vi "Modbus Master Example.vi"() -> ()   [LabVIEW 2018]
doc: "An example of the modbus master functionality."
uses:
  API/Wrapper/API Main.lvlib
  Master Function Definition/Read Device ID code.ctl
  Data Model/Device Data Model.lvclass
  API/Wrapper/Create TCP Master.vi
  API/Master/Modbus Master.lvclass
panel:
  out "element":refnum<vi>
  in  "index":i32
  in  "Stop Button":bool
  in  "Port":u16=502
  in  "Set Holding Registers":bool
  in  "Set Coils":bool
  in  "Fetch Discrete Inputs":bool
  in  "Fetch Input Registers":bool
  in  "Fetch Basic Objects":bool
  out "Basic Objects":string[](array[string])
  out "Status":string
  in  "Disconnect":bool
  in  "Connect":bool
  in  "Holding Registers":u16[](array[numeric])=[0, 0, 0, 0, 0, 0, 0, 0]
  out "Input Registers":u16[](array[numeric])
  in  "Coils":bool[](array[boolean])=[FALSE, FALSE, FALSE, FALSE, FALSE, FALSE, FALSE, FALSE]
  out "Discrete Inputs":bool[](array[boolean])
  in  "Slave Address":string="localhost"
  # "Coils are the boolean outputs of a modbus device. This example allows you to set the first 8 outputs."
  # "Holding Registers are the integer outputs of a modbus device. This example allows you to set the first 8 outputs."
  # "Modbus devices can also store objects in their memory, which are variable length strings. This example requests the basic level of objects."
  # "Discrete inputs are the boolean inputs of a modbus device. This example allows you to read the first 8 inputs."
  # "Input Registers are the integer inputs of a modbus device. This example allows you to read the first 8 inputs."
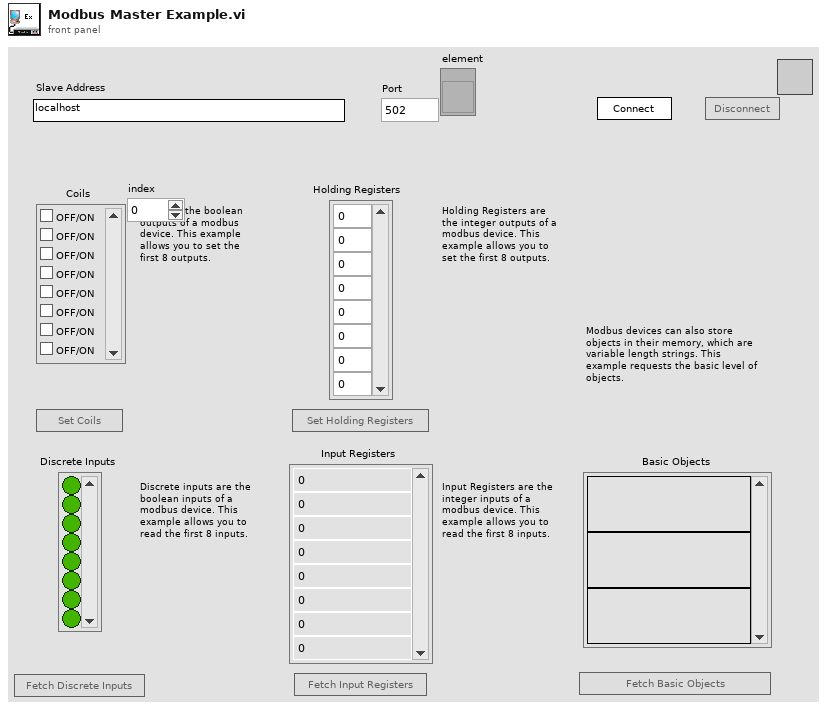
[diagram p1: front panel]
types:
  T1 = enum8{"Enabled", "Disabled", "Disabled and Grayed Out"}
  T2 = typedef "Device Data Model.lvclass/Read Device ID code.ctl" = enum8{"Read Basic", "Read Regular", "Read Extended", "Read Specific"}
  T3 = typedef "Device Data Model.lvclass/Identification Parameters.ctl" = cluster{"Object ID":u8, "Value":string}
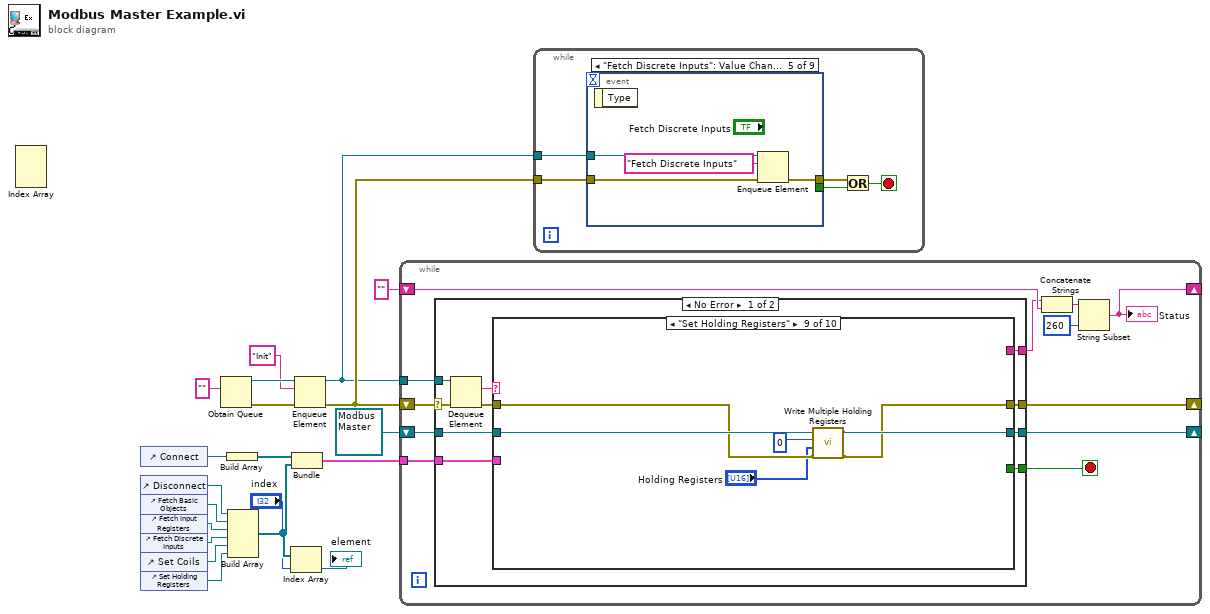
[diagram p0: block diagram]
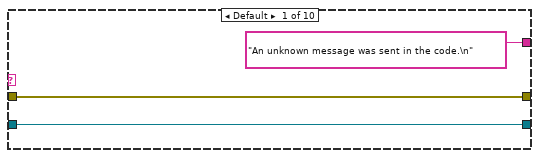
[diagram p2: hidden frame]
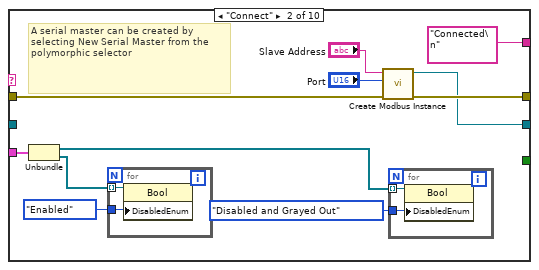
[diagram p3: hidden frame]
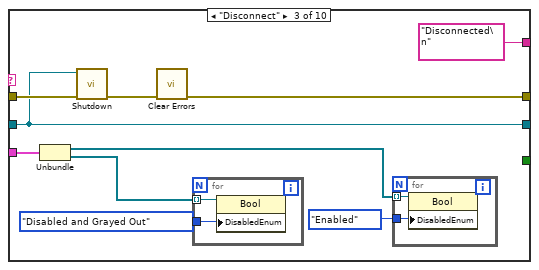
[diagram p4: hidden frame]
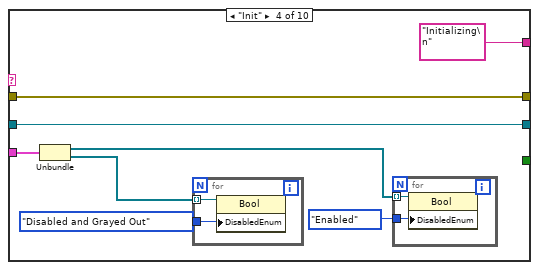
[diagram p5: hidden frame]
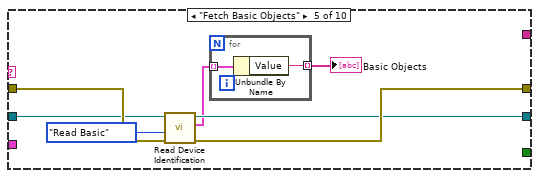
[diagram p6: hidden frame]
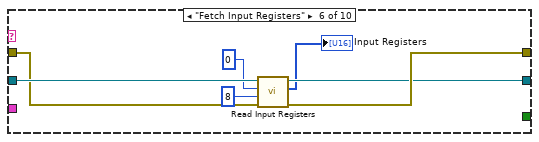
[diagram p7: hidden frame]
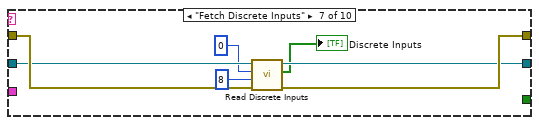
[diagram p8: hidden frame]
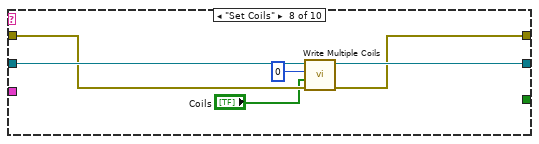
[diagram p9: hidden frame]
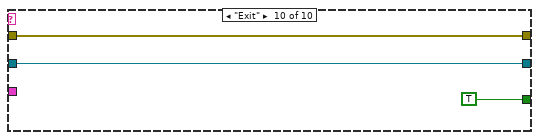
[diagram p10: hidden frame]
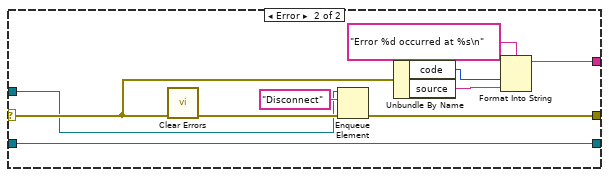
[diagram p11: hidden frame]
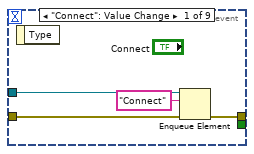
[diagram p12: hidden frame]
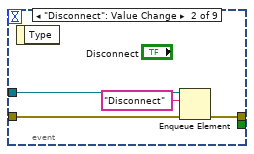
[diagram p13: hidden frame]
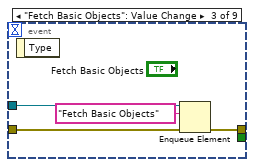
[diagram p14: hidden frame]
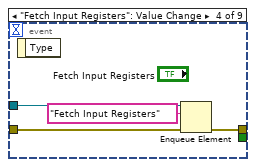
[diagram p15: hidden frame]
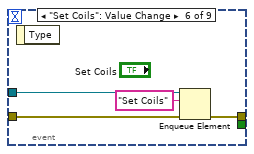
[diagram p16: hidden frame]
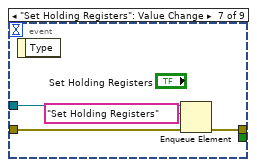
[diagram p17: hidden frame]
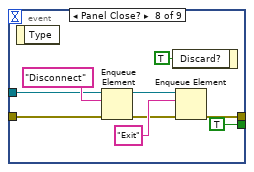
[diagram p18: hidden frame]
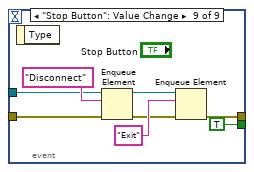
[diagram p19: hidden frame]
diagram:
  n1 = Index Array() -> ()  [unwired: 4 in, 3 out]
  n2 = control-ref of="Connect"() -> (w11:refnum<vi>)
  n3 = control-ref of="Disconnect"() -> (w17:refnum<vi>)
  n4 = control-ref of="Fetch Basic Objects"() -> (w16:refnum<vi>)
  n5 = control-ref of="Fetch Input Registers"() -> (w15:refnum<vi>)
  n6 = control-ref of="Fetch Discrete Inputs"() -> (w14:refnum<vi>)
  n7 = control-ref of="Set Coils"() -> (w13:refnum<vi>)
  n8 = control-ref of="Set Holding Registers"() -> (w12:refnum<vi>)
  n9 = Obtain Queue(element data type="") -> (queue out=w7:refnum<queue>, error out=w20:errorcluster)  [unwired: 4 in, 1 out]
  n10 = Build Array(w11) -> (w9:refnum<vi>[])
  n11 = Build Array(w17, w16, w15, w14, w13, w12) -> (w3:refnum<vi>[])
  n12 = Index Array(array=w3, index="index") -> (element=→"element":refnum<vi>)
  n13 = Bundle(w9, w3) -> (w10:cluster{refnum<vi>[], refnum<vi>[]})  [unwired: 1 in]
  n14 = Enqueue Element(queue=w7, element="Init", error in (no error)=w20) -> (queue out=w6:refnum<queue>, error out=w8:errorcluster)  [unwired: 1 in, 1 out]
  n15 = while {
    shift-right: [w24] -> _
    shift-left: refnum<class "Modbus Master.lvclass"> refnum ("Modbus Master") -> [w23]
    tunnel: w6 -> [w32]
    shift-right: [w30] -> _
    shift-left: w8 -> [w31]
    shift-right: [w29] -> _
    shift-left: "" ("Status") -> [w26]
    tunnel: w10 -> [w21]
    stop <- w22 stop-if-true
    n16 = case shown="No Error" w31 {
      selector: w31 -> [w41 w132]
      tunnel: w32 -> [w42 w126]
      tunnel: [w38 w133] -> w30
      tunnel: [w35 w129] -> w25
      tunnel: [w37 w125] -> w24
      tunnel: w23 -> [w36 w125]
      tunnel: [w34 _] -> w22
      tunnel: w21 -> [w33 _]
      frame No Error {
        n17 = Dequeue Element(queue=w42, error in (no error)=w41) -> (element=w39:string, error out=w40:errorcluster)  [unwired: 1 in, 2 out]
        n18 = case shown="\"Set Holding Registers\"" w39 {
          tunnel: w40 -> [w45 w55 w70 w82 w93 w99 w109 w112 w118 w124]
          tunnel: [w45 w54 w66 w82 w92 w102 w108 w113 w119 w124] -> w38
          tunnel: [w44 w53 w68 w81 w90 w101 w106 w114 w120 w123] -> w37
          tunnel: w36 -> [w44 _ w68 w81 w91 w100 w107 w115 w121 w123]
          tunnel: ["An unknown message was sent in the code.\n" "Connected\n" "Disconnected\n" "Initializing\n" _ _ _ _ _ _] -> w35
          tunnel: [_ _ _ _ _ _ _ _ _ TRUE] -> w34
          tunnel: w33 -> [_ w51 w65 w79 _ _ _ _ _ _]
          frame Default {
          }
          frame "Connect" {
            # "A serial master can be created by selecting New Serial Master from the polymorphic selector"
            n19 = Unbundle(w51) -> (w49:refnum<vi>[], w50:refnum<vi>[])
            n20 = for {
              tunnel: w50 -> [w58] mode=indexing
              tunnel: T1."Enabled" ("Disabled") -> [w57]
              n21 = property class="Bool"(reference=w58, "DisabledEnum"=w57) -> ()  [unwired: 1 in, 2 out]
            }
            n22 = call-poly "Create Modbus Instance.vi"("error in"=w55, "port (502)"="Port", "address"="Slave Address") -> ("error out"=w54:errorcluster, "TCP master instance"=w53:refnum<class "Modbus Master.lvclass">)  [unwired: 7 in]
            n23 = for {
              tunnel: w49 -> [w60] mode=indexing
              tunnel: T1."Disabled and Grayed Out" ("Disabled") -> [w59]
              n24 = property class="Bool"(reference=w60, "DisabledEnum"=w59) -> ()  [unwired: 1 in, 2 out]
            }
          }
          frame "Disconnect" {
            n25 = Unbundle(w65) -> (w63:refnum<vi>[], w64:refnum<vi>[])
            n26 = call-dynamic "Shutdown.vi"("error in"=w70, "Modbus master in"=w68) -> ("error out"=w69:errorcluster)  [unwired: 9 in]
            n27 = call <vilib>:"Clear Errors.vi"("error in (no error)"=w69) -> ("error out"=w66:errorcluster)  [unwired: 5 in, 1 out]
            n28 = for {
              tunnel: w64 -> [w74] mode=indexing
              tunnel: T1."Disabled and Grayed Out" ("Disabled") -> [w73]
              n29 = property class="Bool"(reference=w74, "DisabledEnum"=w73) -> ()  [unwired: 1 in, 2 out]
            }
            n30 = for {
              tunnel: w63 -> [w72] mode=indexing
              tunnel: T1."Enabled" ("Disabled") -> [w71]
              n31 = property class="Bool"(reference=w72, "DisabledEnum"=w71) -> ()  [unwired: 1 in, 2 out]
            }
          }
          frame "Init" {
            n32 = Unbundle(w79) -> (w77:refnum<vi>[], w78:refnum<vi>[])
            n33 = for {
              tunnel: w78 -> [w86] mode=indexing
              tunnel: T1."Disabled and Grayed Out" ("Disabled") -> [w85]
              n34 = property class="Bool"(reference=w86, "DisabledEnum"=w85) -> ()  [unwired: 1 in, 2 out]
            }
            n35 = for {
              tunnel: w77 -> [w84] mode=indexing
              tunnel: T1."Enabled" ("Disabled") -> [w83]
              n36 = property class="Bool"(reference=w84, "DisabledEnum"=w83) -> ()  [unwired: 1 in, 2 out]
            }
          }
          frame "Fetch Basic Objects" {
            n37 = call-dynamic "Read Device Identification.vi"("error in"=w93, "read device ID code"=Read_Device_ID_code."Read Basic" ("Read Device ID code"), "Modbus master in"=w91) -> ("error out"=w92:errorcluster, "objects"=w88:T3[], "Modbus master out"=w90:refnum<class "Modbus Master.lvclass">)  [unwired: 6 in]
            n38 = for {
              tunnel: w88 -> [w95] mode=indexing
              tunnel: [w94] -> w87 mode=indexing
              n39 = Unbundle By Name(w95) -> ("Value"=w94:string)
            }
            "Basic Objects" <- w87
          }
          frame "Fetch Input Registers" {
            n40 = call-dynamic "Read Input Registers.vi"("error in"=w99, "number of inputs"=u16 8 ("number of registers"), "starting address"=u16 0, "Modbus master in"=w100) -> ("error out"=w102:errorcluster, "register values"=→"Input Registers":u16[], "Modbus master out"=w101:refnum<class "Modbus Master.lvclass">)  [unwired: 5 in]
          }
          frame "Fetch Discrete Inputs" {
            n41 = call-dynamic "Read Discrete Inputs.vi"("error in"=w109, "number of inputs"=u16 8, "starting address"=u16 0, "Modbus master in"=w107) -> ("error out"=w108:errorcluster, "discrete inputs"=→"Discrete Inputs":bool[], "Modbus master out"=w106:refnum<class "Modbus Master.lvclass">)  [unwired: 5 in]
          }
          frame "Set Coils" {
            n42 = call-dynamic "Write Multiple Coils.vi"("error in"=w112, "coils to write"="Coils", "starting address"=u16 0, "Modbus master in"=w115) -> ("error out"=w113:errorcluster, "Modbus master out"=w114:refnum<class "Modbus Master.lvclass">)  [unwired: 6 in]
          }
          frame "Set Holding Registers" {
            n43 = call-dynamic "Write Multiple Holding Registers.vi"("error in"=w118, "registers to write"="Holding Registers", "starting address"=u16 0, "Modbus master in"=w121) -> ("error out"=w119:errorcluster, "Modbus master out"=w120:refnum<class "Modbus Master.lvclass">)  [unwired: 6 in]
          }
          frame "Exit" {
          }
        }
      }
      frame Error {
        n44 = call <vilib>:"Clear Errors.vi"("error in (no error)"=w132) -> ("error out"=w134:errorcluster)  [unwired: 5 in, 1 out]
        n45 = Enqueue Element(queue=w126, element="Disconnect", error in (no error)=w134) -> (error out=w133:errorcluster)  [unwired: 1 in, 2 out]
        n46 = Unbundle By Name(w132) -> ("code"=w131:i32, "source"=w130:string)
        n47 = Format Into String(format string="Error %d occurred at %s\n", w131, w130) -> (resulting string=w129:string)  [unwired: 2 in, 1 out]
      }
    }
    n48 = Concatenate Strings(w25, w26) -> (w27:string)
    n49 = String Subset(string=w27, length (rest)=260 ("length (rest)")) -> (substring=w29:string)  [unwired: 1 in]
    "Status" <- w29
  }
  n50 = while {
    tunnel: w8 -> [w139]
    tunnel: w6 -> [w138]
    stop <- w135 stop-if-true
    n51 = event shown="[4] \"Fetch Discrete Inputs\": Value Change" {
      selector: _ -> [_ _ _ _ _ _ _ _ _]
      dyn-events: _ -> [_ _ _ _ _ _ _ _ _]
      timeout: _ -> [_ _ _ _ _ _ _ _ _]
      tunnel: w139 -> [w143 w147 w151 w155 w159 w163 w167 w173 w182]
      tunnel: [w142 w146 w150 w154 w158 w162 w166 w168 w177] -> w137
      tunnel: w138 -> [w141 w145 w149 w153 w157 w161 w165 w170 w179]
      tunnel: [_ _ _ _ _ _ _ TRUE ("Discard?") TRUE ("Discard?")] -> w136
      event "Connect": Value Change {
        n52 = event-data() -> ()  [unwired: 1 in, 1 out]
        n53 = Enqueue Element(queue=w141, element="Connect", error in (no error)=w143) -> (error out=w142:errorcluster)  [unwired: 1 in, 2 out]
      }
      event "Disconnect": Value Change {
        n54 = event-data() -> ()  [unwired: 1 in, 1 out]
        n55 = Enqueue Element(queue=w145, element="Disconnect", error in (no error)=w147) -> (error out=w146:errorcluster)  [unwired: 1 in, 2 out]
      }
      event "Fetch Basic Objects": Value Change {
        n56 = event-data() -> ()  [unwired: 1 in, 1 out]
        n57 = Enqueue Element(queue=w149, element="Fetch Basic Objects", error in (no error)=w151) -> (error out=w150:errorcluster)  [unwired: 1 in, 2 out]
      }
      event "Fetch Input Registers": Value Change {
        n58 = event-data() -> ()  [unwired: 1 in, 1 out]
        n59 = Enqueue Element(queue=w153, element="Fetch Input Registers", error in (no error)=w155) -> (error out=w154:errorcluster)  [unwired: 1 in, 2 out]
      }
      event "Fetch Discrete Inputs": Value Change {
        n60 = event-data() -> ()  [unwired: 1 in, 1 out]
        n61 = Enqueue Element(queue=w157, element="Fetch Discrete Inputs", error in (no error)=w159) -> (error out=w158:errorcluster)  [unwired: 1 in, 2 out]
      }
      event "Set Coils": Value Change {
        n62 = event-data() -> ()  [unwired: 1 in, 1 out]
        n63 = Enqueue Element(queue=w161, element="Set Coils", error in (no error)=w163) -> (error out=w162:errorcluster)  [unwired: 1 in, 2 out]
      }
      event "Set Holding Registers": Value Change {
        n64 = event-data() -> ()  [unwired: 1 in, 1 out]
        n65 = Enqueue Element(queue=w165, element="Set Holding Registers", error in (no error)=w167) -> (error out=w166:errorcluster)  [unwired: 1 in, 2 out]
      }
      event Panel Close? {
        n66 = event-data() -> ()  [unwired: 1 in, 1 out]
        n67 = Enqueue Element(queue=w170, element="Disconnect", error in (no error)=w173) -> (queue out=w171:refnum<queue>, error out=w169:errorcluster)  [unwired: 1 in, 1 out]
        n68 = event-data("Discard?"=TRUE) -> ()  [unwired: 1 in, 1 out]
        n69 = Enqueue Element(queue=w171, element="Exit", error in (no error)=w169) -> (error out=w168:errorcluster)  [unwired: 1 in, 2 out]
      }
      event "Stop Button": Value Change {
        n70 = event-data() -> ()  [unwired: 1 in, 1 out]
        n71 = Enqueue Element(queue=w179, element="Disconnect", error in (no error)=w182) -> (queue out=w180:refnum<queue>, error out=w178:errorcluster)  [unwired: 1 in, 1 out]
        n72 = Enqueue Element(queue=w180, element="Exit", error in (no error)=w178) -> (error out=w177:errorcluster)  [unwired: 1 in, 2 out]
      }
    }
    n73 = Or(x=w137, y=w136) -> (x .or. y?=w135:bool)
  }
